vi "工控机端口检查.vi"() -> ()   [LabVIEW 2013]
panel:
  in  "stop":bool
  out "消息":string
  in  "Check":bool
  in  "油压":T1(ring)
  in  "行程":T1(ring)
  # "行程"
  # "油压"
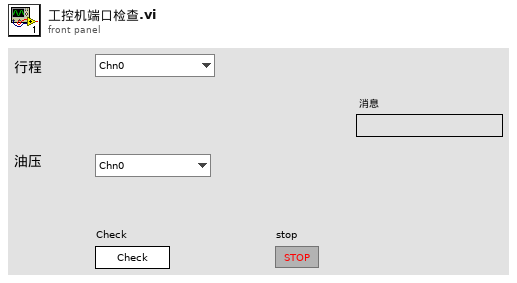
[diagram p1: front panel]
types:
  T1 = enum16{"Chn0", "Chn1", "Chn2", "Chn3", "Chn4", "Chn5"}
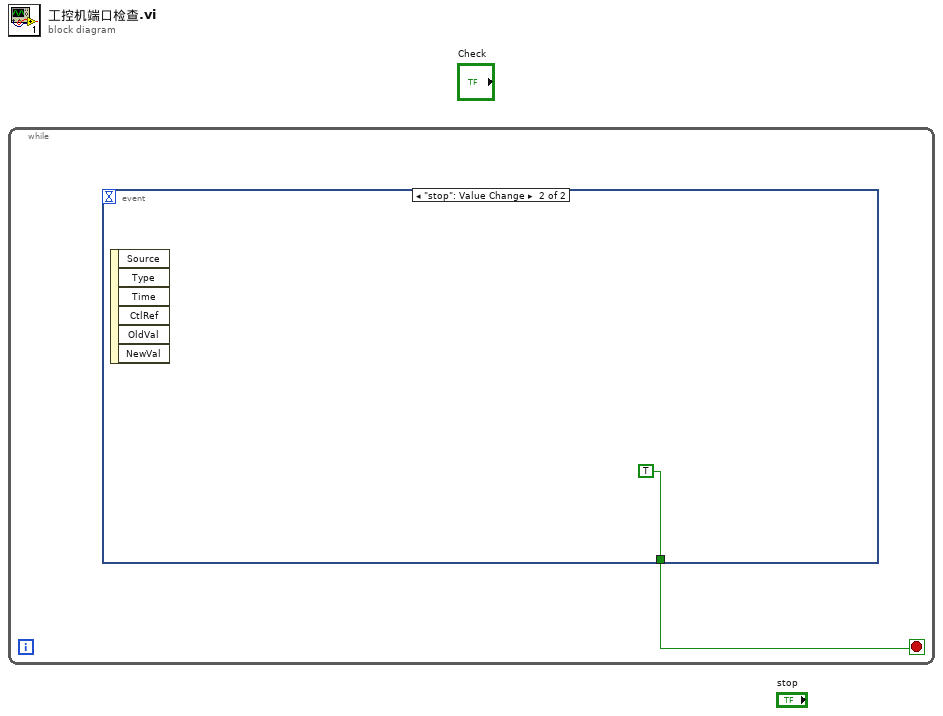
[diagram p0: block diagram]
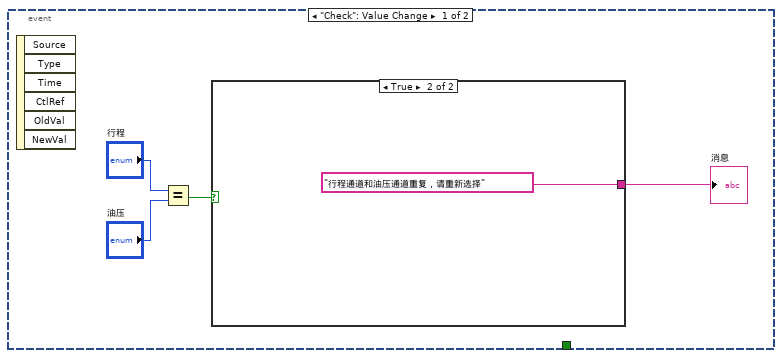
[diagram p2: hidden frame]
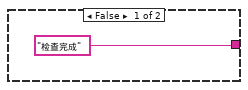
[diagram p3: hidden frame]
diagram:
  n1 = while {
    stop <- w1 stop-if-true
    n2 = event shown="[1] \"stop\": Value Change" {
      selector: _ -> [_ _]
      dyn-events: _ -> [_ _]
      timeout: _ -> [_ _]
      tunnel: [_ TRUE] -> w1
      event "Check": Value Change {
        n3 = event-data() -> ()  [unwired: 1 in, 6 out]
        n4 = Equal?(x="行程", y="油压") -> (x = y?=w3:bool)
        n5 = case shown="True" w3 {
          tunnel: ["检查完成" "行程通道和油压通道重复，请重新选择"] -> w2
          frame False {
          }
          frame True {
          }
        }
        "消息" <- w2
      }
      event "stop": Value Change {
        n6 = event-data() -> ()  [unwired: 1 in, 6 out]
      }
    }
  }
